vi "Helmholtz2D_FEM_Init Data.vi"(0 "F(x, y)":dbl[](array[numeric]), 1 "Grid":cluster{"Xi":dbl[], "Yi":dbl[]}, 5 "k":dbl=1.0, 7 "a":dbl, 9 "Domain":cluster{"X":dbl[], "Y":dbl[]}, 12 "Boundary Condition":cluster{"type":T3, "Value":dbl[]} {"type" items=["Dirichlet", "Neumann"]}) -> (4 "Helmholtz2D FEM Data":T1)   [LabVIEW 2017, in "NI_PDE.lvlib"]
uses:
  <vilib>/gmath/NI_PDE.lvlib
  <vilib>/gmath/pde.llb/Common/PDE_BC Type.ctl
  <vilib>/gmath/pde.llb/Helmholtz2D_FEM/Helmholtz2D_FEM_Data.ctl
  <vilib>/gmath/pde.llb/Common/PDE_Sparse Mtrx.ctl
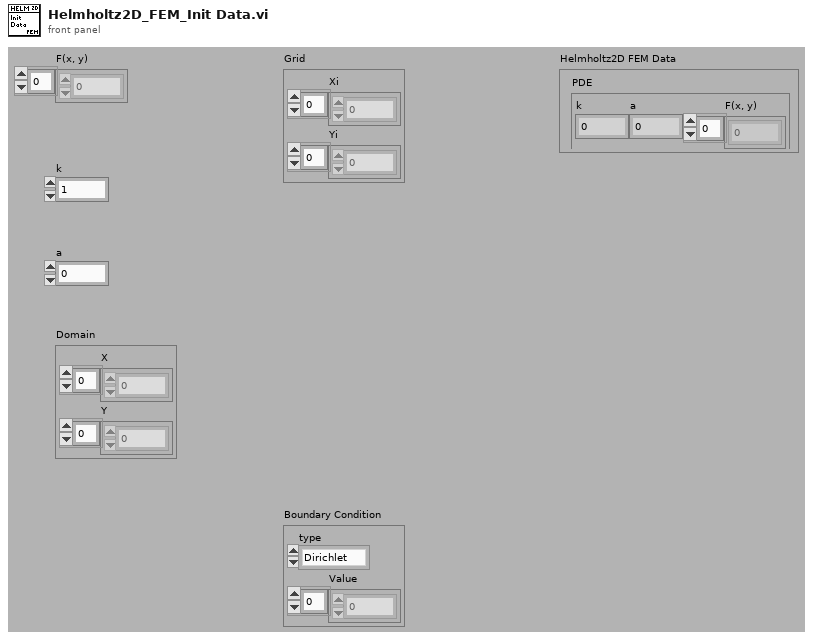
[diagram p1: front panel]
types:
  T1 = typedef "NI_PDE.lvlib/Helmholtz2D_FEM_Data.ctl" = cluster{"PDE":cluster{"k":dbl, "a":dbl, "F(x, y)":dbl[]}, "# of unknown":i32, "# of known":i32, "U(x, y)":dbl[], "X Used":dbl[], "Y Used":dbl[], "Triangulation":i32[][], "Coef Mtrx":T2}
  T2 = typedef "NI_PDE.lvlib/PDE_Sparse Mtrx.ctl" = cluster{"Row":cluster{"col":i32, "value":dbl}[]}[]
  T3 = typedef "NI_PDE.lvlib/PDE_BC Type.ctl" = i32
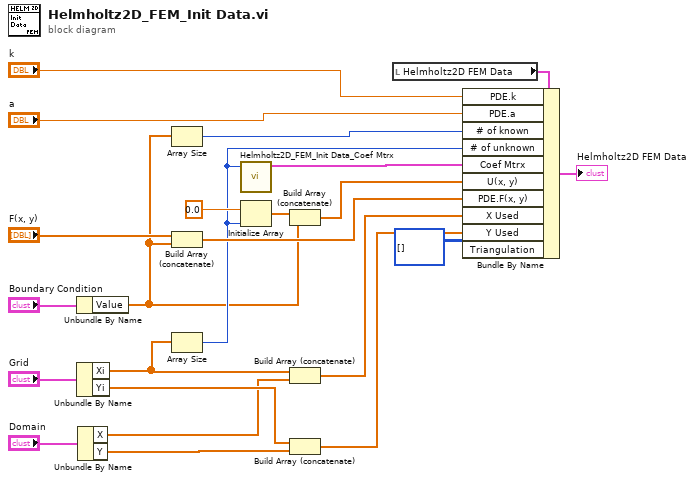
[diagram p0: block diagram]
diagram:
  n1 = Unbundle By Name("Boundary Condition") -> ("Value"=w1:dbl[])
  n2 = Unbundle By Name("Grid") -> ("Xi"=w4:dbl[], "Yi"=w7:dbl[])
  n3 = Unbundle By Name("Domain") -> ("X"=w6:dbl[], "Y"=w5:dbl[])
  n4 = Array Size(array=w1) -> (size(s)=w2:i32)
  n5 = Build Array (concatenate)("F(x, y)", w1) -> (w15:dbl[])
  n6 = Array Size(array=w4) -> (size(s)=w3:i32)
  n7 = call <vilib>:"Helmholtz2D_FEM_Init Data_Coef Mtrx.vi"("# of unknown"=w3) -> ("Coef Mtrx"=w16:T2)  [unwired: 10 out]
  n8 = Initialize Array(0.0 ("element"), w3) -> (w13:dbl[])
  n9 = Build Array (concatenate)(w13, w1) -> (w12:dbl[])
  n10 = Build Array (concatenate)(w4, w6) -> (w11:dbl[])
  n11 = Build Array (concatenate)(w7, w5) -> (w10:dbl[])
  n12 = local read "Helmholtz2D FEM Data"() -> (w23:T1)
  n13 = Bundle By Name(cluster=w23, "PDE.k"="k", "PDE.a"="a", "# of known"=w2, "# of unknown"=w3, "Coef Mtrx"=w16, "U(x, y)"=w12, "PDE.F(x, y)"=w15, "X Used"=w11, "Y Used"=w10, "Triangulation"=i32[][] [] ("Triangluation")) -> (→"Helmholtz2D FEM Data":T1)
